vi "xt.vi"(10 "stages":T2[](array[typedef]) {"t (s)" format="%#_6e"; "v_i (m/s)" format="%#_6e"; "a (m / s^2)" format="%#_6e"; "d (m)" format="%#_6e"; "v_f (m/s)" format="%#_6e"}, 11 "dt (s)":dbl=1e-08 format="%#_6p") -> (2 "output":T1, 3 "num_steps":i32)   [LabVIEW 2017, in "wf.lvlib" / "wf_tools.lvlib"]
uses:
  wf_tools.lvlib
  stage.ctl
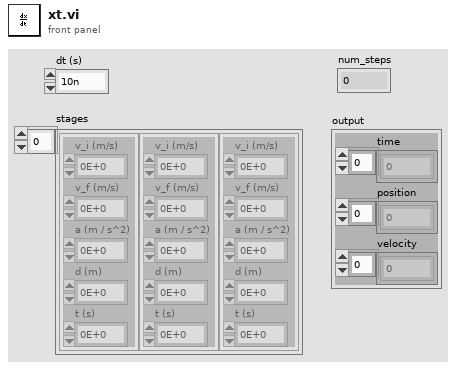
[diagram p1: front panel]
types:
  T1 = cluster{"time":dbl[], "position":dbl[], "velocity":dbl[]}
  T2 = typedef "wf.lvlib/wf_tools.lvlib/stage.ctl" = cluster{"v_i (m/s)":dbl, "v_f (m/s)":dbl, "a (m / s^2)":dbl, "d (m)":dbl, "t (s)":dbl}
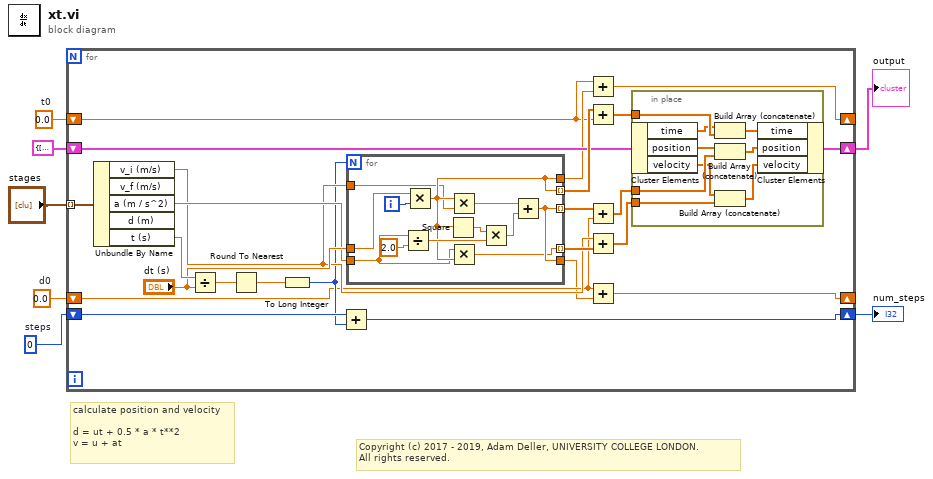
[diagram p0: block diagram]
diagram:
  w3 = 0  # steps
  w5 = 0.0  # d0
  w7 = 0.0  # t0
  # "Copyright (c) 2017 - 2019, Adam Deller, UNIVERSITY COLLEGE LONDON.\nAll rights reserved."
  # "calculate position and velocity\n\nd = ut + 0.5 * a * t**2\nv = u + at"
  n1 = for {
    shift-right: [w12] -> _
    shift-left: w7 -> [w11]
    tunnel: "stages" -> [w31] mode=indexing
    shift-right: [w8] -> _
    shift-left: w5 -> [w10]
    shift-right: [w18] -> w1
    shift-left: T1 {"time"=[], "position"=[], "velocity"=[]} ("trap") -> [w19]
    shift-right: [w14] -> w2
    shift-left: w3 -> [w16]
    n2 = Unbundle By Name(w31) -> ("v_i (m/s)"=w17:dbl, "a (m / s^2)"=w26:dbl, "t (s)"=w30:dbl)  [unwired: 2 out]
    n3 = Divide(x=w30, y="dt (s)") -> (x/y=w29:dbl)
    n4 = Round To Nearest(number=w29) -> (nearest integer value=w28:dbl)
    n5 = To Long Integer(number=w28) -> (32bit integer=w15:i32)
    n6 = Add(x=w16, y=w15) -> (x+y=w14:i32)
    n7 = for {
      N: w15 -> [_]
      tunnel: [w45] -> w24 mode=indexing
      tunnel: [w44] -> w25 mode=indexing
      tunnel: "dt (s)" -> [w46]
      tunnel: w26 -> [w43]
      tunnel: [w45] -> w9
      tunnel: [w44] -> w13
      tunnel: [w42] -> w22 mode=indexing
      tunnel: w17 -> [w41]
      i -> [w52]
      n8 = Divide(x=w43, y=2.0) -> (x/y=w49:dbl)
      n9 = Multiply(x=w46, y=w52) -> (x*y=w44:dbl)
      n10 = Square(x=w44) -> (x^2=w48:dbl)
      n11 = Multiply(x=w44, y=w41) -> (x*y=w50:dbl)
      n12 = Multiply(x=w43, y=w44) -> (x*y=w42:dbl)
      n13 = Multiply(x=w48, y=w49) -> (x*y=w47:dbl)
      n14 = Add(x=w50, y=w47) -> (x+y=w45:dbl)
    }
    n15 = Add(x=w11, y=w13) -> (x+y=w12:dbl)
    n16 = Add(x=w25, y=w11) -> (x+y=w21:dbl[])
    n17 = Add(x=w24, y=w10) -> (x+y=w23:dbl[])
    n18 = Add(x=w17, y=w22) -> (x+y=w20:dbl[])
    n19 = Add(x=w10, y=w9) -> (x+y=w8:dbl)
    n20 = in-place {
      in-place-border: w23 -> [w40]
      in-place-border: w21 -> [w39]
      in-place-border: w20 -> [w38]
      n21 = in-place-cluster #1(w19) -> ("time"=w37:dbl[], "position"=w35:dbl[], "velocity"=w33:dbl[])
      n22 = Build Array (concatenate)(w37, w39) -> (w36:dbl[])
      n23 = Build Array (concatenate)(w35, w40) -> (w34:dbl[])
      n24 = Build Array (concatenate)(w33, w38) -> (w32:dbl[])
      n25 = in-place-cluster #1("time"=w36, "position"=w34, "velocity"=w32) -> (w18:T1)
    }
  }
  "output" <- w1
  "num_steps" <- w2
